vi "niScope Configure Trigger Window.vi"(0 "instrument handle":refnum<k15>, 1 "trigger window mode":T3, 2 "trigger coupling":T2=1 items=["AC"=0, "DC"=1, "HF Reject"=3, "LF Reject"=4, "AC Plus HF Reject"=1001], 5 "trigger source":T1="0" caption="trigger source (Channel 0)", 7 "low level":dbl format="%.2f", 9 "high level":dbl format="%.2f", 11 "error in":errorcluster, 12 "trigger holdoff":dbl format="%.4f", 13 "trigger delay":dbl format="%.4f") -> (4 "instrument handle out":refnum<k15>, 15 "error out":errorcluster)   [LabVIEW 2013]
doc: "Configures common properties for window triggering. A window trigger occurs when a signal enters or leaves a window you specify with the <B>high level</B> or <B>low level</B> parameters."
uses:
  <instrlib>/niScope/Controls/niScope trigger window mode.ctl
  <instrlib>/niScope/Controls/niScope trigger coupling.ctl
  <instrlib>/niScope/Controls/niScope trigger source.ctl
  niScope_32.dll
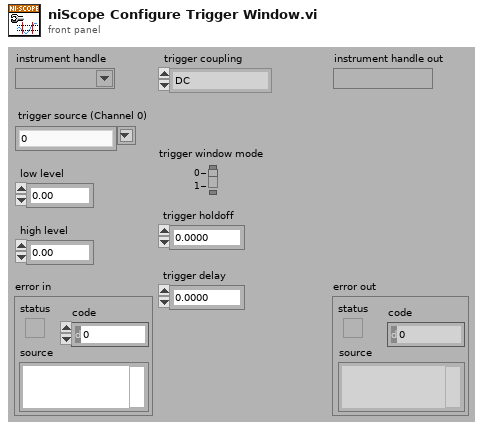
[diagram p1: front panel]
types:
  T1 = typedef "niScope trigger source.ctl" = string
  T2 = typedef "niScope trigger coupling.ctl" = u16
  T3 = typedef "niScope trigger window mode.ctl" = i32
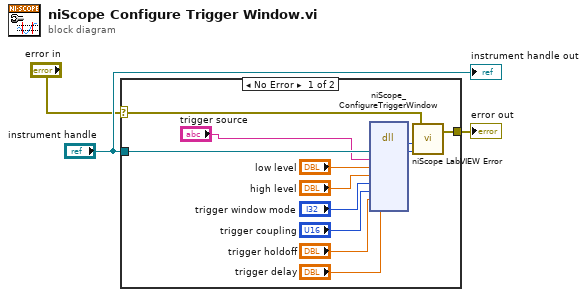
[diagram p0: block diagram]
diagram:
  n1 = case shown="No Error" "error in" {
    selector: "error in" -> [w5 w16]
    tunnel: [w12 w16] -> w3
    tunnel: "instrument handle" -> [w15 _]
    frame No Error {
      n2 = dll-call lib="niScope_*.*" fn="niScope_ConfigureTriggerWindow"("instrument handle"=w15, "triggerSource"="trigger source", "lowLevel"="low level", "highLevel"="high level", "windowMode"="trigger window mode", "coupling"="trigger coupling", "holdoff"="trigger holdoff", "delay"="trigger delay") -> ("status"=w14:i32, "instrument handle"=w13:u32)  [unwired: 10 in, 2 out]
      n3 = call <instrlib>:"niScope LabVIEW Error.vi"("instrument handle"=w13, "niScope error code (0)"=w14, "error in (no error)"=w5) -> ("error out"=w12:errorcluster)  [unwired: 2 in]
    }
    frame Error {
    }
  }
  "error out" <- w3
  "instrument handle out" <- "instrument handle"
